vi "Set Meas Step Name.vi"(8 "error in (no error)":errorcluster, 10 "Step In":refnum<k7>, 11 "SPECAN_IQSLOT in":refnum<class "SPECAN_IQSLOT.lvclass">) -> (0 "error out":errorcluster, 2 "Step Out":refnum<k7>, 3 "SPECAN_IQSLOT out":refnum<class "SPECAN_IQSLOT.lvclass">)   [LabVIEW 2018, in "SPECAN_IQSLOT.lvlib" / "SPECAN_IQSLOT.lvclass"]
uses:
  SPECAN_IQSLOT.lvclass
  C:/Sequence Automation/Plugins/Measurement Interface.lvlibp/Measurement Interface.lvclass
  Plugins/Measurement Interface.lvlibp/Private Methods/Measurement Name/Read Measurement Name.vi
  Plugins/TestStand API Tools (TSAT).lvlibp/Step Actions/TSAT Step Actions.lvlib
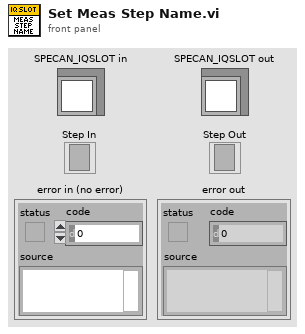
[diagram p1: front panel]
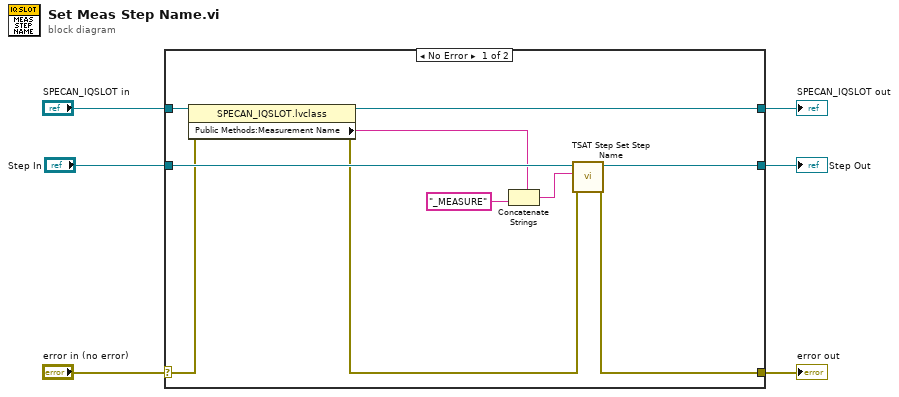
[diagram p0: block diagram]
diagram:
  n1 = case shown="No Error" "error in (no error)" {
    selector: "error in (no error)" -> [w12 w19]
    tunnel: [w10 w19] -> w5
    tunnel: [w15 w18] -> w3
    tunnel: "SPECAN_IQSLOT in" -> [w16 w18]
    tunnel: "Step In" -> [w14 w17]
    tunnel: [w13 w17] -> w1
    frame No Error {
      n2 = property class="SPECAN_IQSLOT.lvclass"(reference=w16, error in=w12) -> (reference out=w15:refnum<class "SPECAN_IQSLOT.lvclass">, error out=w11:errorcluster, "Public Methods:Measurement Name"=w7:string)
      n3 = Concatenate Strings(w7, "_MEASURE" ("Name")) -> (w8:string)
      n4 = call "TSAT Step Set Step Name.vi"("Error In"=w11, "Name"=w8, "Step In"=w14) -> ("Error Out"=w10:errorcluster, "Step Out"=w13:refnum<k7>)  [unwired: 7 in]
    }
    frame Error {
    }
  }
  "error out" <- w5
  "SPECAN_IQSLOT out" <- w3
  "Step Out" <- w1
